vi "3.90.1-Grab Shutdown Queue.vi"() -> (0 "queue out":refnum<queue>)   [LabVIEW 2010]
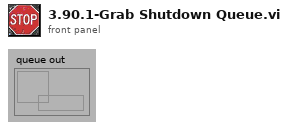
[diagram p1: front panel]
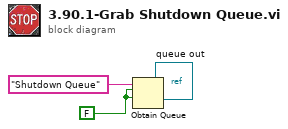
[diagram p0: block diagram]
diagram:
  w1 = FALSE
  n1 = Obtain Queue(name (unnamed)="Shutdown Queue", element data type=w1, create if not found? (T)=w1) -> (queue out=→"queue out":refnum<queue>)  [unwired: 2 in, 2 out]
